vi "transition.vi"(8 "error in (no error)":errorcluster, 10 "ContextData In":refnum<class "ContextData.lvclass">, 11 "Initialize in":refnum<class "Launch UI.lvclass">) -> (0 "error out":errorcluster, 2 "ContextData Out":refnum<class "ContextData.lvclass">, 3 "Next State":refnum<class "State.lvclass">)   [LabVIEW 2019, in "Launch UI.lvclass"]
uses:
  Launch UI.lvclass
  ContextData/ContextData.lvclass
  State/State.lvclass
  Welcome/Welcome.lvclass
  C:/Users/fflores/Documents/GitHub Projects/Simon/Simon Game/OOP States/State/State.lvclass
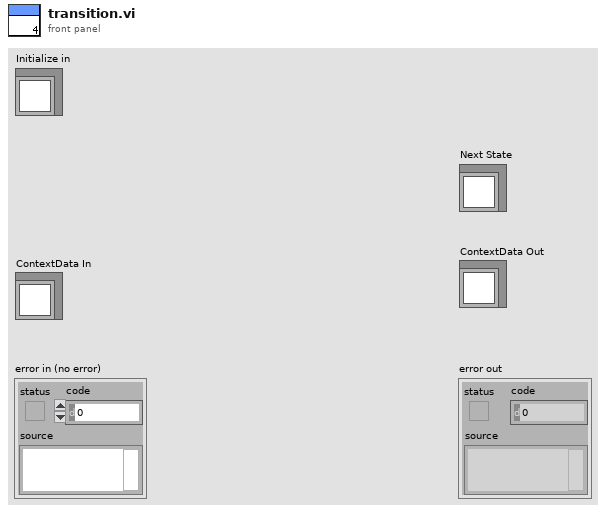
[diagram p1: front panel]
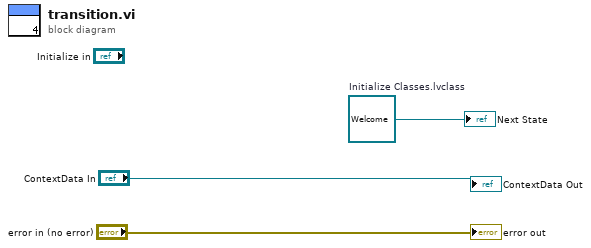
[diagram p0: block diagram]
diagram:
  w1 = refnum<class "Welcome.lvclass"> refnum  # Initialize Classes.lvclass
  "error out" <- "error in (no error)"
  "ContextData Out" <- "ContextData In"
  "Next State" <- w1
